vi "Get Data Frame.vi"(8 "error in":errorcluster, 10 "Unit ID (A)":string="A", 11 "VISA Session In":refnum<visa-resource-name>="Alicat") -> (0 "error out":errorcluster, 2 "Returned Data Frame":string, 3 "VISA Session Out":refnum<visa-resource-name>)   [LabVIEW 2019]
doc: "Polls the Alicat device for data and returns the Alicat's un-edited data string (space delimited)."
uses:
  <vilib>/Instr/_visa.llb/VISA Flush IO Buffer Mask.ctl
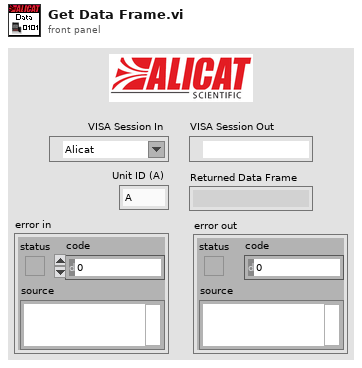
[diagram p1: front panel]
types:
  T1 = typedef "VISA Flush IO Buffer Mask.ctl" = u16
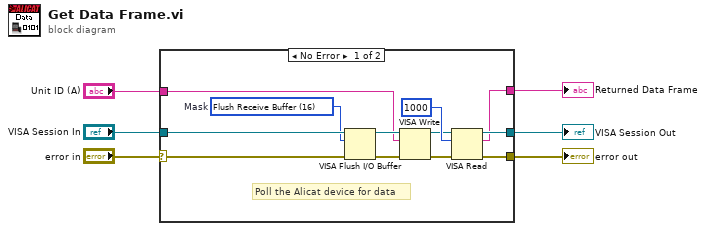
[diagram p0: block diagram]
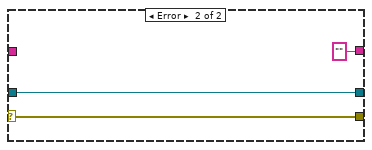
[diagram p2: hidden frame]
diagram:
  n1 = case shown="No Error" "error in" {
    selector: "error in" -> [w12 w20]
    tunnel: "VISA Session In" -> [w13 w21]
    tunnel: "Unit ID (A)" -> [w10 _]
    tunnel: [w8 w21] -> w3
    tunnel: [w9 w20] -> w2
    tunnel: [w7 "" ("read buffer")] -> w1
    frame No Error {
      w11 = T1 16 items=["Flush Receive Buffer"=16, "Write Transmit Buffer to Device"=32, "Flush Receive Buffer (No I/O)"=64, "Flush Transmit Buffer"=128]  # Mask
      # "Poll the Alicat device for data"
      n2 = VISA Flush I/O Buffer(VISA resource name=w13, mask (16)=w11, error in (no error)=w12) -> (VISA resource name out=w15:refnum<visa-resource-name>, error out=w17:errorcluster)
      n3 = VISA Write(VISA resource name=w15, write buffer=w10, error in (no error)=w17) -> (VISA resource name out=w14:refnum<visa-resource-name>, error out=w16:errorcluster)  [unwired: 1 out]
      n4 = VISA Read(VISA resource name=w14, byte count=u32 1000, error in (no error)=w16) -> (VISA resource name out=w8:refnum<visa-resource-name>, read buffer=w7:string, error out=w9:errorcluster)  [unwired: 1 out]
    }
    frame Error {
    }
  }
  "error out" <- w2
  "VISA Session Out" <- w3
  "Returned Data Frame" <- w1
